vi "Datacluster manually remove bad data pts.vi"(10 "Datasets to be processed":T2(array[cluster]), 11 "data cluster":cluster{"all rows":dbl[][]}[](array[cluster])) -> (3 "data cluster out":cluster{"all rows":dbl[][]}[](array[cluster]))   [LabVIEW 2021]
panel:
  in  "selected XY data":dbl[][](array[numeric])
  in  "operation":enum16{"keep pts", "delete pts", "move pts"}(ring)=enum."delete pts"
  in  "start over":bool
  in  "auto scale once":bool
  in  "Do not Save and Proceed":bool
  in  "reset cursors":bool
  out "String":string="KR6_Rh3In3Ge4"
  in  "Undo":bool
  in  "Save and Proceed":bool
  in  "data selection mode":T1(ring)
  in  "Update":bool
  out "XY Graph":cluster{"x-array":dbl[], "y-array":dbl[]}(graph)
  # "Caution: All rows will be affected."
  # "Operation\ndelete/keep data pts: selected data pts will be removed or kept.\nmove data pts: (1) use zoom/drag selection mode (2) type in data"
  # "Remove pts"
  # "(4) Start processing"
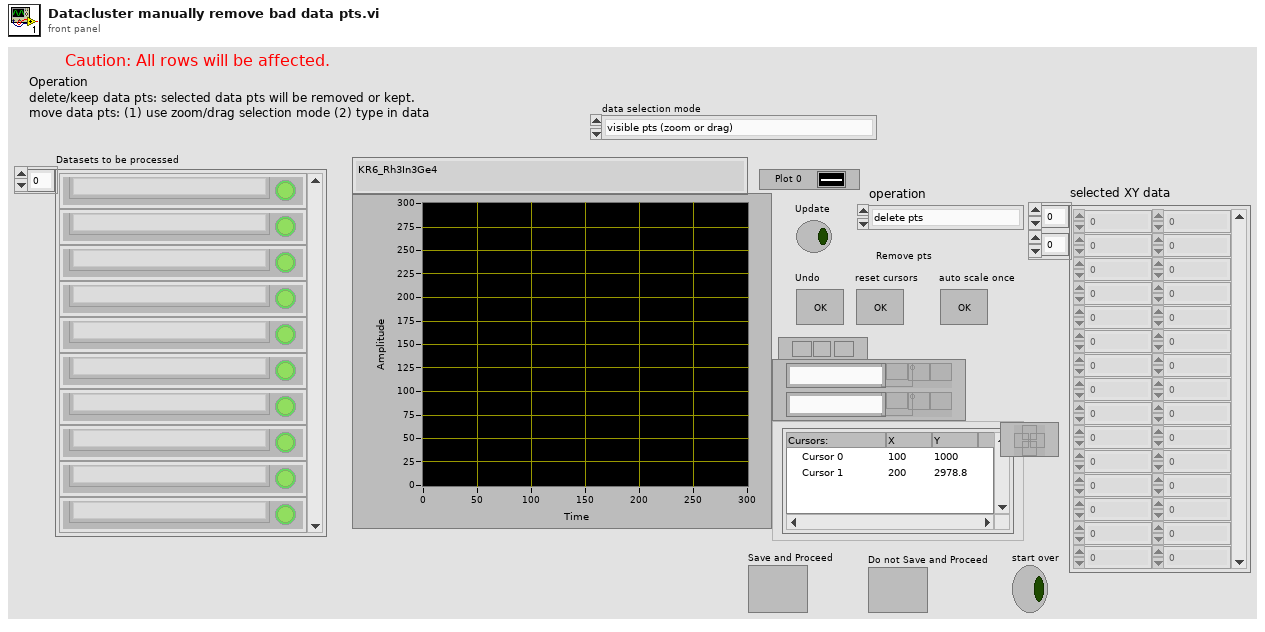
[diagram p1: front panel]
types:
  T1 = enum16{"visible pts (zoom or drag)", "pts inside the rectangle defined by the cursors", "pts between two horizontal cursors", "pts between two vertical cursor lines"}
  T2 = cluster{"String":string, "Boolean":bool, "begin":u32, "length":u32, "y weight":dbl}[]
  T3 = enum16{"no change", "show whole data", "show whole panel"}
  T4 = enum16{"no change", "no auto", "auto once", "auto"}
  T5 = enum16{"no change", "move to data center", "move to data corner", "move to panel center", "move to panel corner"}
  T6 = enum16{"no change", "hide cursor", "cross", "horizontal", "vertical"}
  T7 = enum16{"visible pts (use zoom or drag)", "pts inside rectangle defined the cursor lines", "pts between two horizontal cursors", "pts between two vertical cursor lines"}
  T8 = typedef "LVCursorListTypeDef.ctl" = cluster{"Name":string, "Color":u32, "Style":u8, "Point Style":u8, "Name Visible":bool, "Allow Drag":bool, "Cursor Mode":u32, "Plot":i32, "Index":i32, "Position":cluster{"X":dbl, "Y":dbl}, "X Scale":u32, "Y Scale":u32, "Watch Plots":i32[], "Watch All Plots":bool, "Plot Area":i32, "Label Offset":cluster{"X":dbl, "Y":dbl}}[]
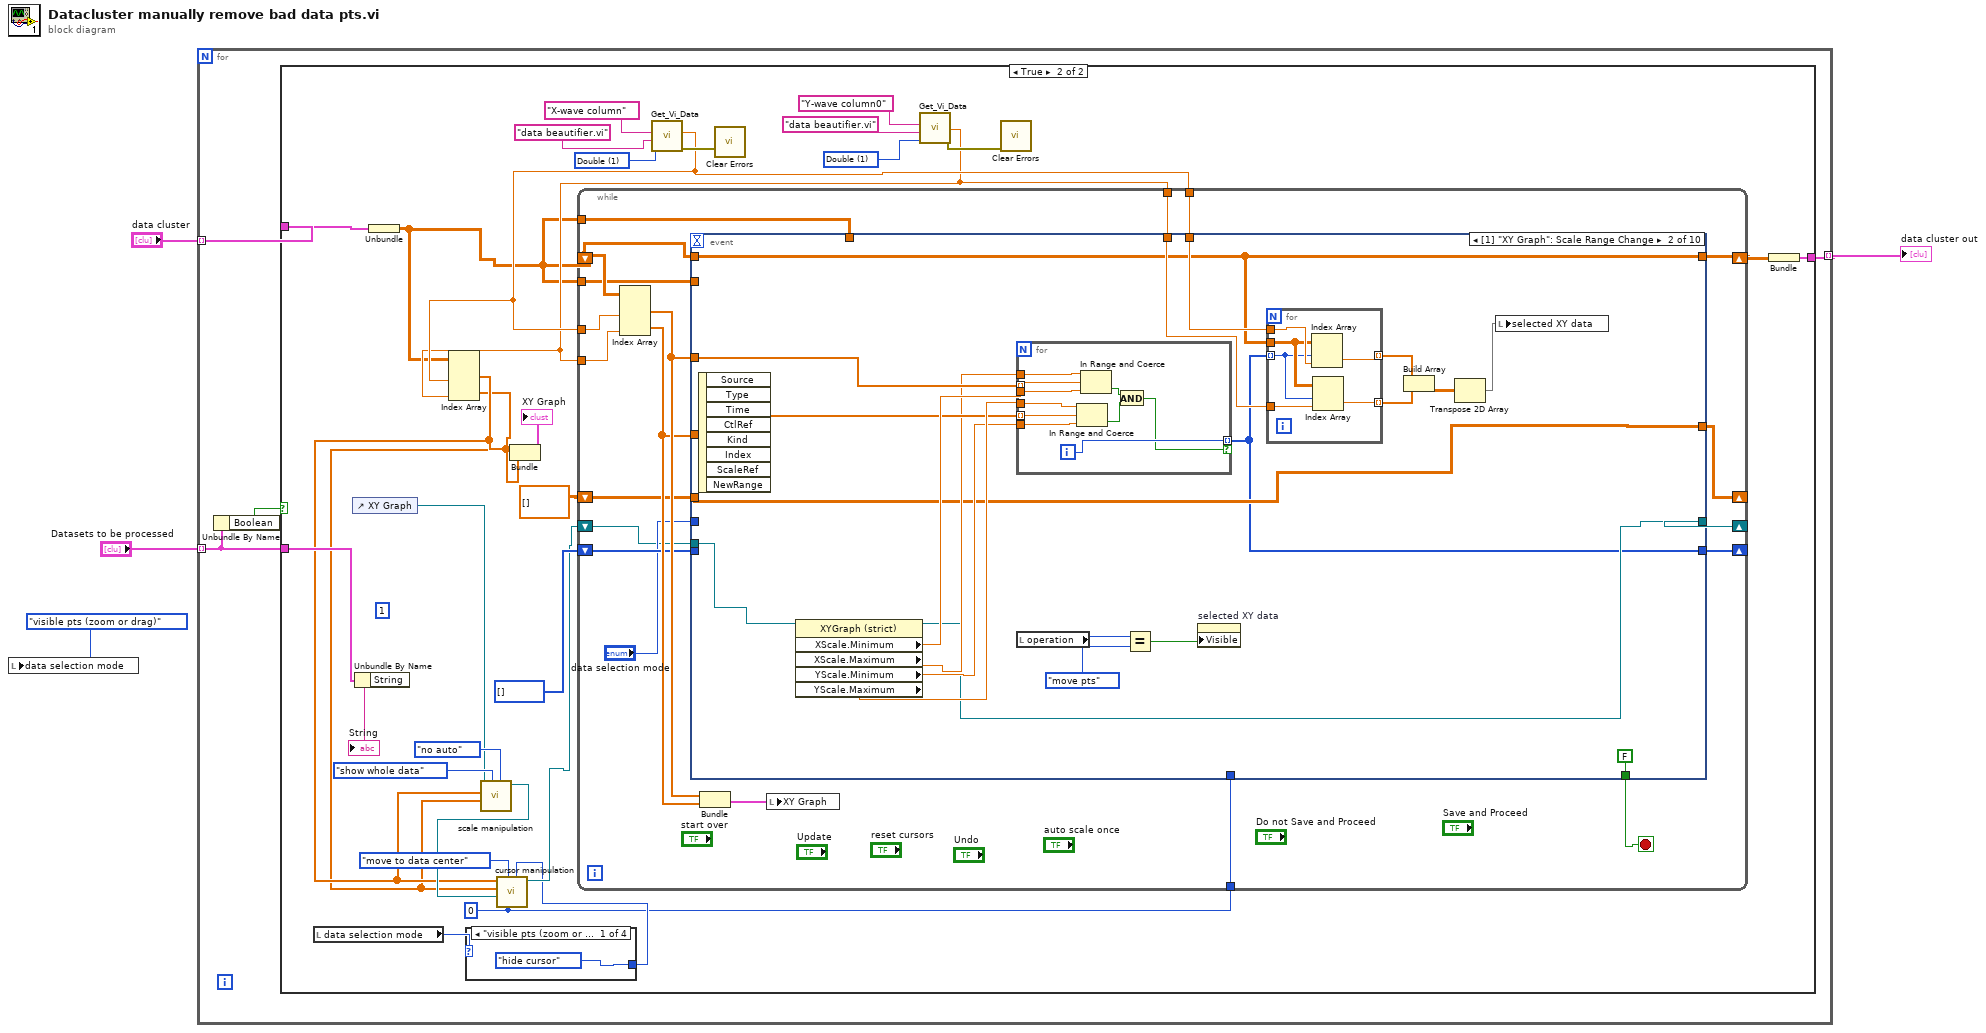
[diagram p0: block diagram]
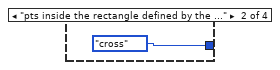
[diagram p3: hidden frame]
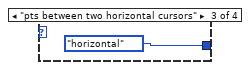
[diagram p4: hidden frame]
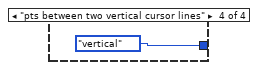
[diagram p5: hidden frame]
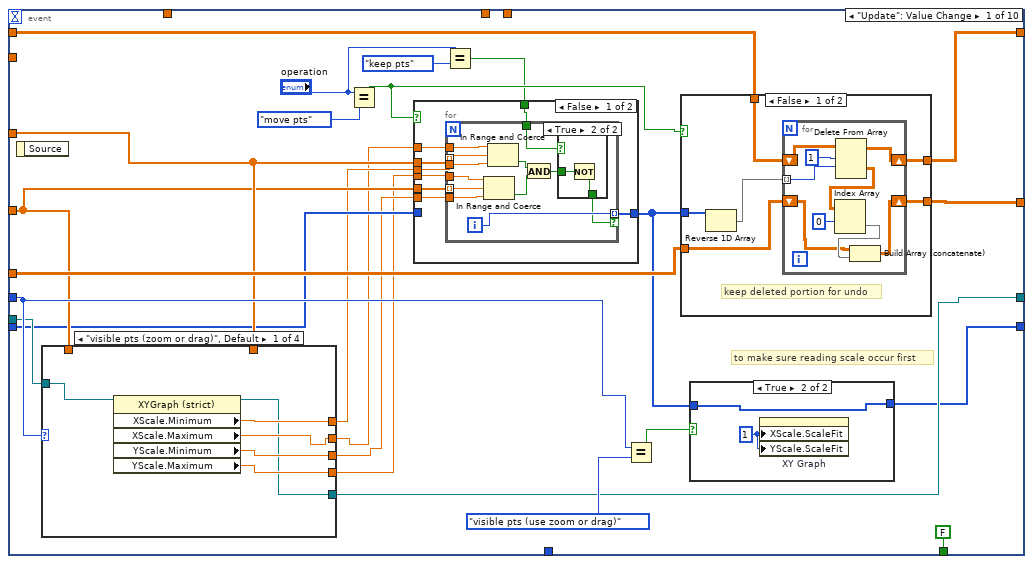
[diagram p6: hidden frame]
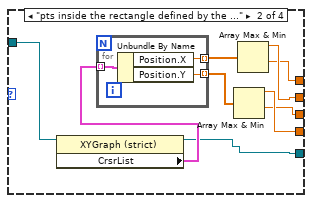
[diagram p11: hidden frame]
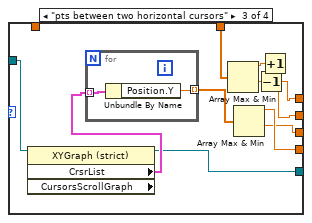
[diagram p12: hidden frame]
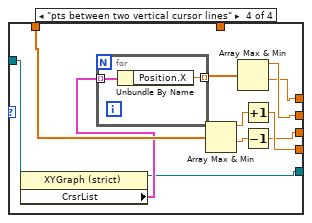
[diagram p13: hidden frame]
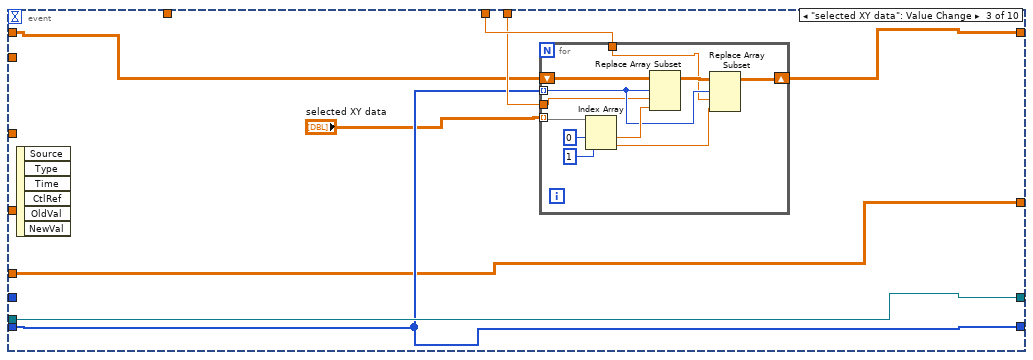
[diagram p14: hidden frame]
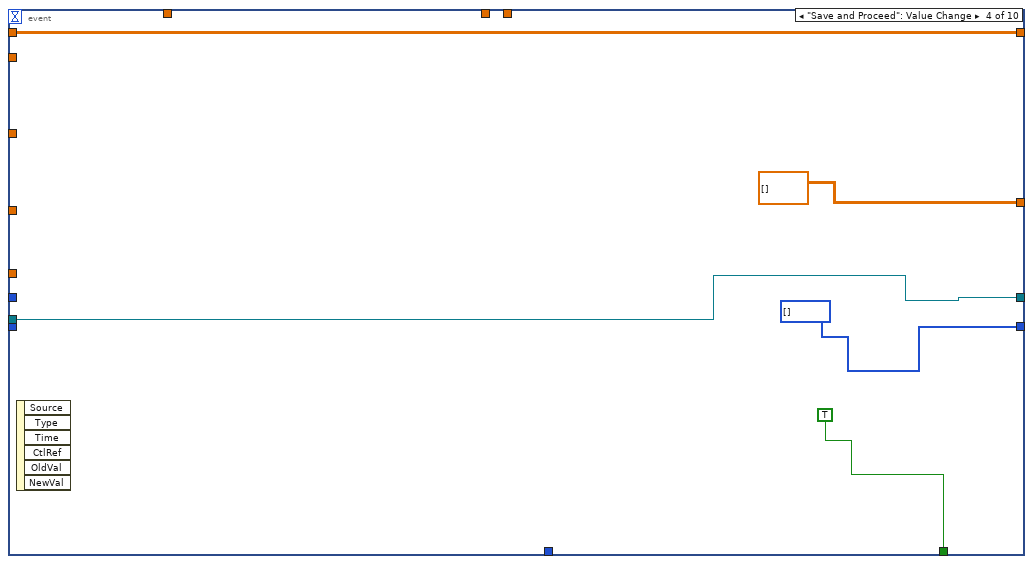
[diagram p15: hidden frame]
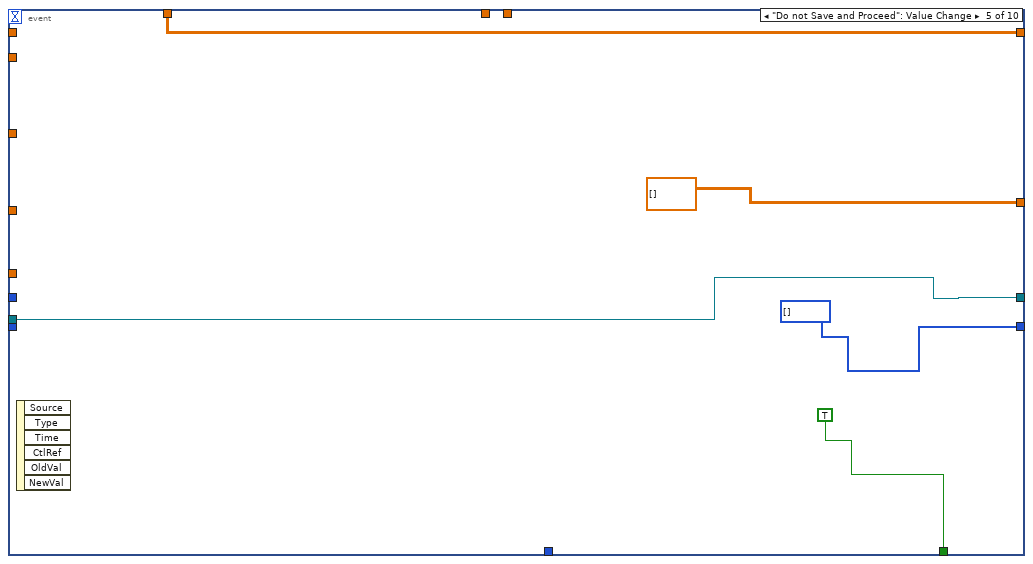
[diagram p16: hidden frame]
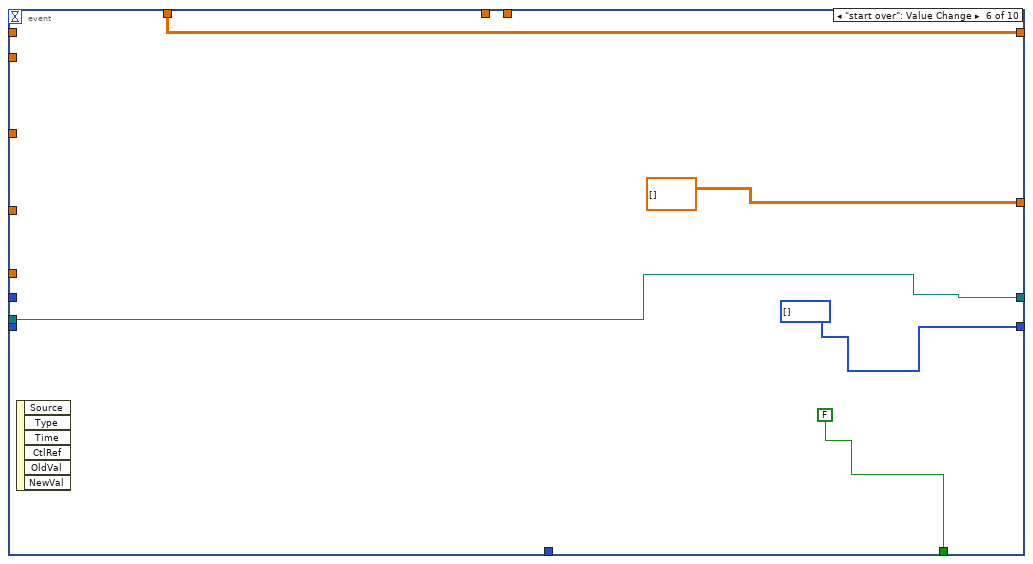
[diagram p17: hidden frame]
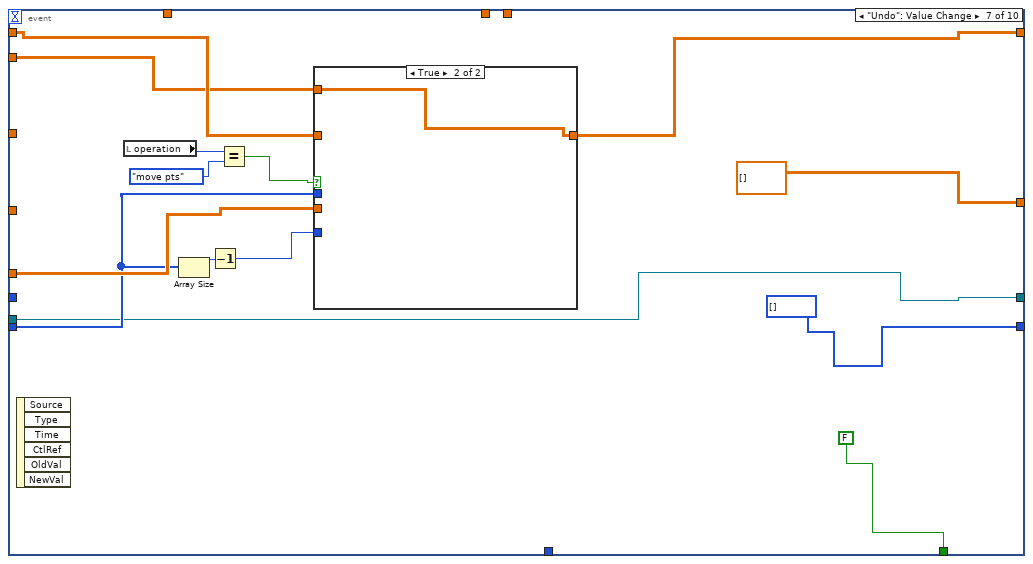
[diagram p18: hidden frame]
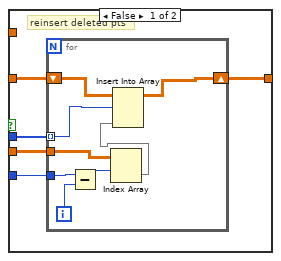
[diagram p19: hidden frame]
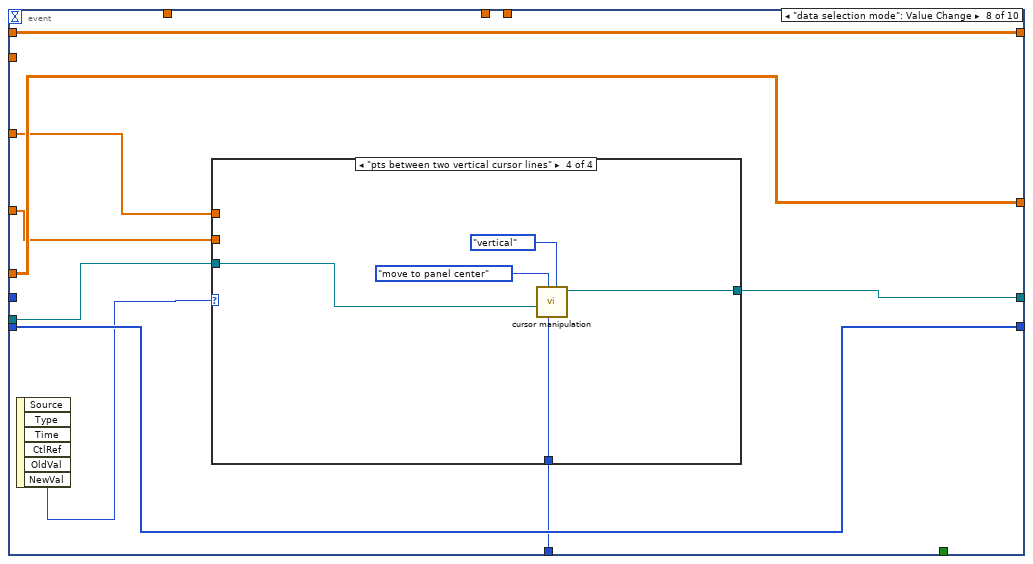
[diagram p20: hidden frame]
diagram:
  n1 = local write "data selection mode"(T1."visible pts (zoom or drag)" ("data selection mode")) -> ()
  n2 = for {
    tunnel: "Datasets to be processed" -> [w6] mode=indexing
    tunnel: "data cluster" -> [w8] mode=indexing
    tunnel: [w7] -> w2 mode=indexing
    n3 = Unbundle By Name(w6) -> ("Boolean"=w5:bool)
    n4 = case shown="True" w5 {
      tunnel: w6 -> [_ w27]
      tunnel: w8 -> [w9 w26]
      tunnel: [w9 w25] -> w7
      frame False {
      }
      frame True {
        w14 = u32 0 ("Cursor.Cursor Mode")
        (unwired) u8 1 ("X Scale.Scale Fit")
        w33 = u16 1 items=["String", "Double", "Boolean", "Variant"] ("Data Type")
        w36 = u16 1 items=["String", "Double", "Boolean", "Variant"] ("Data Type")
        n5 = local read "data selection mode"() -> (w16:T1)
        n6 = control-ref of="XY Graph"() -> (w17:refnum<vi>)
        n7 = Unbundle By Name(w27) -> ("String"=→"String":string)
        n8 = Unbundle(w26) -> ("all rows"=w10:dbl[][])
        n9 = case shown="\"visible pts (zoom or drag)\", Default" w16 {
          tunnel: [T6."hide cursor" ("cursor type") T6."cross" ("cursor type") T6."horizontal" ("cursor type") T6."vertical" ("cursor type")] -> w15
          frame "visible pts (zoom or drag)", Default {
          }
          frame "pts inside the rectangle defined by the cursors" {
          }
          frame "pts between two horizontal cursors" {
          }
          frame "pts between two vertical cursor lines" {
          }
        }
        n10 = call "Get_Vi_Data.vi"("Data Type"=w36, "VI name"="data beautifier.vi", "Control Name"="X-wave column") -> ("error out"=w35:errorcluster, "Data (Double)"=w12:dbl)  [unwired: 4 in, 3 out]
        n11 = call <vilib>:"Clear Errors.vi"("error in (no error)"=w35) -> ()  [unwired: 5 in, 2 out]
        n12 = call "Get_Vi_Data.vi"("Data Type"=w33, "VI name"="data beautifier.vi", "Control Name"="Y-wave column0") -> ("error out"=w31:errorcluster, "Data (Double)"=w11:dbl)  [unwired: 4 in, 3 out]
        n13 = Index Array(array=w10, index (col) #1=w12, index (col) #2=w11) -> (element #1=w19:dbl[], element #2=w18:dbl[])  [unwired: 2 in]
        n14 = call "scale manipulation.vi"("scale fit"=T4."no auto", "rescale"=T3."show whole data", "y-array"=w18, "x-array"=w19, "graph reference in"=w17) -> ("reference out"=w22:refnum<vi>)  [unwired: 6 in]
        n15 = call "cursor manipulation.vi"("cursor type"=w15, "Cursor.Cursor Mode"=w14, "cursor position"=T5."move to data center" ("mode"), "graph reference in"=w22, "y-array"=w18, "x-array"=w19) -> ("reference out"=w21:refnum<vi>)  [unwired: 5 in]
        n16 = Bundle("all rows"=w19, "all rows"=w18) -> (→"XY Graph":cluster{"all rows":dbl[], "all rows":dbl[]})  [unwired: 1 in]
        n17 = while {
          tunnel: w12 -> [w47]
          tunnel: w11 -> [w54]
          shift-right: [w60] -> w39
          shift-left: w10 -> [w61]
          shift-right: [w57] -> _
          shift-left: dbl[][] [] -> [w58]
          shift-right: [w56] -> _
          shift-left: i32[] [] -> [w55]
          tunnel: w10 -> [w52]
          tunnel: w14 -> [w49]
          shift-right: [w48] -> _
          shift-left: w21 -> [w51]
          tunnel: w12 -> [w46]
          tunnel: w11 -> [w45]
          tunnel: w10 -> [w44]
          stop <- w59 stop-if-true
          n18 = Index Array(array=w61, index (col) #1=w47, index (col) #2=w54) -> (element #1=w63:dbl[], element #2=w62:dbl[])  [unwired: 2 in]
          n19 = event shown="[1] \"XY Graph\": Scale Range Change" {
            selector: _ -> [_ _ _ _ _ _ _ _ _ _]
            dyn-events: _ -> [_ _ _ _ _ _ _ _ _ _]
            timeout: _ -> [_ _ _ _ _ _ _ _ _ _]
            tunnel: w63 -> [w79 w192 _ _ _ _ _ w279 _ w314]
            tunnel: w62 -> [w78 w191 _ _ _ _ _ w278 _ w313]
            tunnel: w61 -> [w87 w183 w215 w236 _ _ w260 w280 w309 w318]
            tunnel: [w86 w183 w218 w236 w239 w244 w254 w280 w309 w318] -> w60
            tunnel: [FALSE FALSE _ TRUE TRUE FALSE FALSE _ _ _] -> w59
            tunnel: [w84 w182 w214 dbl[][] [] dbl[][] [] dbl[][] [] dbl[][] [] w283 w311 w320] -> w57
            tunnel: w58 -> [w83 w182 w214 _ _ _ w259 w283 w311 w320]
            tunnel: [w65 w180 w216 i32[] [] i32[] [] i32[] [] i32[] [] w282 w310 w319] -> w56
            tunnel: w55 -> [w70 _ w216 _ _ _ w257 w282 w310 w319]
            tunnel: "data selection mode" -> [w82 _ _ _ _ _ _ _ _ _]
            tunnel: w52 -> [_ _ _ _ w239 w244 _ _ _ _]
            tunnel: w51 -> [w72 w189 w217 w232 w237 w242 w251 w277 w308 w317]
            tunnel: w49 -> [_ _ _ _ _ _ _ w276 w305 _]
            tunnel: [w71 w188 w217 w232 w237 w242 w251 w275 w304 w312] -> w48
            tunnel: w46 -> [_ w187 w219 _ _ _ _ _ _ _]
            tunnel: w45 -> [_ w186 w220 _ _ _ _ _ _ _]
            tunnel: w44 -> [_ _ _ _ _ _ w247 _ _ _]
            event "Update": Value Change {
              # "to make sure reading scale occur first"
              n20 = event-data() -> ()  [unwired: 1 in, 1 out]
              n21 = case shown="\"visible pts (zoom or drag)\", Default" w82 {
                tunnel: [w133 w142 w157 w167] -> w66
                tunnel: [w134 w141 w156 w166] -> w67
                tunnel: [w136 w143 w153 w171] -> w69
                tunnel: [w135 w144 w154 w172] -> w68
                tunnel: w79 -> [_ _ w155 _]
                tunnel: w78 -> [_ _ _ w168]
                tunnel: w72 -> [w137 w140 w152 w165]
                tunnel: [w132 w138 w150 w163] -> w71
                frame "visible pts (zoom or drag)", Default {
                  n22 = property class="XYGraph (strict)"(reference=w137) -> (reference out=w132:refnum<vi>, "XScale.Minimum"=w136:dbl, "XScale.Maximum"=w135:dbl, "YScale.Minimum"=w134:dbl, "YScale.Maximum"=w133:dbl)  [unwired: 1 in, 1 out]
                }
                frame "pts inside the rectangle defined by the cursors" {
                  n23 = property class="XYGraph (strict)"(reference=w140) -> (reference out=w138:refnum<vi>, "CrsrList"=w139:T8)  [unwired: 1 in, 1 out]
                  n24 = for {
                    tunnel: w139 -> [w149] mode=indexing
                    tunnel: [w148] -> w146 mode=indexing
                    tunnel: [w147] -> w145 mode=indexing
                    n25 = Unbundle By Name(w149) -> ("Position.X"=w148:dbl, "Position.Y"=w147:dbl)
                  }
                  n26 = Array Max & Min(array=w145) -> (max value=w142:dbl, min value=w141:dbl)  [unwired: 2 out]
                  n27 = Array Max & Min(array=w146) -> (max value=w144:dbl, min value=w143:dbl)  [unwired: 2 out]
                }
                frame "pts between two horizontal cursors" {
                  n28 = property class="XYGraph (strict)" props=["CrsrList", "CursorsScrollGraph"](reference=w152) -> (reference out=w150:refnum<vi>, "CrsrList"=w151:T8)  [unwired: 1 in, 2 out]
                  n29 = for {
                    tunnel: [w162] -> w160 mode=indexing
                    tunnel: w151 -> [w161] mode=indexing
                    n30 = Unbundle By Name(w161) -> ("Position.Y"=w162:dbl)
                  }
                  n31 = Array Max & Min(array=w155) -> (max value=w159:dbl, min value=w158:dbl)  [unwired: 2 out]
                  n32 = Array Max & Min(array=w160) -> (max value=w157:dbl, min value=w156:dbl)  [unwired: 2 out]
                  n33 = Decrement(x=w158) -> (x-1=w153:dbl)
                  n34 = Increment(x=w159) -> (x+1=w154:dbl)
                }
                frame "pts between two vertical cursor lines" {
                  n35 = property class="XYGraph (strict)"(reference=w165) -> (reference out=w163:refnum<vi>, "CrsrList"=w164:T8)  [unwired: 1 in, 1 out]
                  n36 = for {
                    tunnel: w164 -> [w175] mode=indexing
                    tunnel: [w174] -> w173 mode=indexing
                    n37 = Unbundle By Name(w175) -> ("Position.X"=w174:dbl)
                  }
                  n38 = Array Max & Min(array=w168) -> (max value=w170:dbl, min value=w169:dbl)  [unwired: 2 out]
                  n39 = Array Max & Min(array=w173) -> (max value=w172:dbl, min value=w171:dbl)  [unwired: 2 out]
                  n40 = Increment(x=w170) -> (x+1=w167:dbl)
                  n41 = Decrement(x=w169) -> (x-1=w166:dbl)
                }
              }
              n42 = Equal?(x="operation", y=enum16{"keep pts", "delete pts", "move pts"}."move pts") -> (x = y?=w76:bool)
              n43 = Equal?(x="operation", y=enum16{"keep pts", "delete pts", "move pts"}."keep pts") -> (x = y?=w73:bool)
              n44 = case shown="False" w76 {
                tunnel: w66 -> [w95 _]
                tunnel: w67 -> [w94 _]
                tunnel: w69 -> [w93 _]
                tunnel: [w92 w111] -> w64
                tunnel: w79 -> [w91 _]
                tunnel: w78 -> [w90 _]
                tunnel: w73 -> [w89 _]
                tunnel: w68 -> [w88 _]
                tunnel: w70 -> [_ w111]
                frame False {
                  n45 = for {
                    tunnel: w91 -> [w107] mode=indexing
                    tunnel: w90 -> [w103] mode=indexing
                    tunnel: w95 -> [w102]
                    tunnel: [w104] -> w92 mode=indexing if=w96
                    tunnel: w94 -> [w101]
                    tunnel: w88 -> [w100]
                    tunnel: w93 -> [w99]
                    tunnel: w89 -> [w98]
                    i -> [w104]
                    n46 = In Range and Coerce(upper limit=w102, x=w103, lower limit=w101) -> (In Range?=w106:bool)  [unwired: 1 out]
                    n47 = In Range and Coerce(upper limit=w100, x=w107, lower limit=w99) -> (In Range?=w105:bool)  [unwired: 1 out]
                    n48 = And(x=w105, y=w106) -> (x .and. y?=w97:bool)
                    n49 = case shown="True" w98 {
                      tunnel: w97 -> [w108 w110]
                      tunnel: [w108 w109] -> w96
                      frame False {
                      }
                      frame True {
                        n50 = Not(x=w110) -> (.not. x?=w109:bool)
                      }
                    }
                  }
                }
                frame True {
                }
              }
              n51 = Equal?(x=w82, y=T7."visible pts (use zoom or drag)") -> (x = y?=w80:bool)
              n52 = case shown="False" w76 {
                tunnel: w87 -> [w117 w128]
                tunnel: [w116 w128] -> w86
                tunnel: [w115 w127] -> w84
                tunnel: w83 -> [w113 w127]
                tunnel: w64 -> [w112 _]
                frame False {
                  # "keep deleted portion for undo"
                  n53 = Reverse 1D Array(array=w112) -> (reversed array=w114:i32[])
                  n54 = for {
                    tunnel: w114 -> [w125] mode=indexing
                    shift-right: [w126] -> w116
                    shift-left: w117 -> [w123]
                    shift-right: [w119] -> w115
                    shift-left: w113 -> [w118]
                    n55 = Delete From Array(array=w123, length=1, index (row)=w125) -> (deleted portion=w122:dbl[][], array with subset deleted=w126:dbl[][])  [unwired: 1 in]
                    n56 = Index Array(array=w122, index (row)=0) -> (element=w120:dbl[])  [unwired: 1 in]
                    n57 = Build Array (concatenate)(w118, w120) -> (w119:dbl[][])
                  }
                }
                frame True {
                }
              }
              n58 = case shown="True" w80 {
                tunnel: [w129 w130] -> w65
                tunnel: w64 -> [w129 w130]
                frame False {
                }
                frame True {
                  w131 = u8 1 ("X Scale.Scale Fit")
                  n59 = property on="XY Graph" class="XYGraph (strict)"("XScale.ScaleFit"=w131, "YScale.ScaleFit"=w131) -> ()  [unwired: 2 in, 2 out]
                }
              }
            }
            event "XY Graph": Scale Range Change {
              n60 = event-data() -> ()  [unwired: 1 in, 8 out]
              n61 = property class="XYGraph (strict)"(reference=w189) -> (reference out=w188:refnum<vi>, "XScale.Minimum"=w194:dbl, "XScale.Maximum"=w190:dbl, "YScale.Minimum"=w195:dbl, "YScale.Maximum"=w196:dbl)  [unwired: 1 in, 1 out]
              n62 = for {
                tunnel: w192 -> [w212] mode=indexing
                tunnel: w191 -> [w208] mode=indexing
                tunnel: w196 -> [w207]
                tunnel: [w209] -> w180 mode=indexing if=w203
                tunnel: w195 -> [w206]
                tunnel: w190 -> [w205]
                tunnel: w194 -> [w204]
                i -> [w209]
                n63 = In Range and Coerce(upper limit=w207, x=w208, lower limit=w206) -> (In Range?=w211:bool)  [unwired: 1 out]
                n64 = In Range and Coerce(upper limit=w205, x=w212, lower limit=w204) -> (In Range?=w210:bool)  [unwired: 1 out]
                n65 = And(x=w210, y=w211) -> (x .and. y?=w203:bool)
              }
              n66 = local read "operation"() -> (w179:enum16{"keep pts", "delete pts", "move pts"})
              n67 = Equal?(x=w179, y=enum16{"keep pts", "delete pts", "move pts"}."move pts" ("operation")) -> (x = y?=w176:bool)
              n68 = property on="selected XY data" class="Arr (strict)"("Visible"=w176) -> ()  [unwired: 2 in, 2 out]
              n69 = for {
                tunnel: w180 -> [w200] mode=indexing
                tunnel: w183 -> [w201]
                tunnel: w187 -> [w202]
                tunnel: w186 -> [w199]
                tunnel: [w198] -> w185 mode=indexing
                tunnel: [w197] -> w184 mode=indexing
                n70 = Index Array(array=w201, index (row)=w200, index (col)=w202) -> (element=w198:dbl)
                n71 = Index Array(array=w201, index (row)=w200, index (col)=w199) -> (element=w197:dbl)
              }
              n72 = Build Array(w185, w184) -> (w181:dbl[][])
              n73 = Transpose 2D Array(2D array=w181) -> (transposed array=w177:dbl[][])
              n74 = local write "selected XY data"(w177) -> ()
            }
            event "selected XY data": Value Change {
              n75 = event-data() -> ()  [unwired: 1 in, 6 out]
              n76 = for {
                tunnel: w216 -> [w225] mode=indexing
                tunnel: w220 -> [w221]
                tunnel: "selected XY data" -> [w230] mode=indexing
                shift-right: [w223] -> w218
                shift-left: w215 -> [w231]
                tunnel: w219 -> [w222]
                n77 = Index Array(array=w230, index #1=0 ("index"), index #2=1 ("index")) -> (element #1=w227:dbl, element #2=w224:dbl)
                n78 = Replace Array Subset(array=w231, new element=w227, index (row)=w225, index (col)=w222) -> (w226:dbl[][])
                n79 = Replace Array Subset(array=w226, new element=w224, index (row)=w225, index (col)=w221) -> (w223:dbl[][])
              }
            }
            event "Save and Proceed": Value Change {
              n80 = event-data() -> ()  [unwired: 1 in, 6 out]
            }
            event "Do not Save and Proceed": Value Change {
              n81 = event-data() -> ()  [unwired: 1 in, 6 out]
            }
            event "start over": Value Change {
              n82 = event-data() -> ()  [unwired: 1 in, 6 out]
            }
            event "Undo": Value Change {
              n83 = event-data() -> ()  [unwired: 1 in, 6 out]
              n84 = local read "operation"() -> (w250:enum16{"keep pts", "delete pts", "move pts"})
              n85 = Array Size(array=w257) -> (size(s)=w258:i32)
              n86 = Decrement(x=w258) -> (x-1=w256:i32)
              n87 = Equal?(x=w250, y=enum16{"keep pts", "delete pts", "move pts"}."move pts" ("operation")) -> (x = y?=w248:bool)
              n88 = case shown="True" w248 {
                tunnel: w260 -> [w265 _]
                tunnel: w259 -> [w264 _]
                tunnel: w257 -> [w263 _]
                tunnel: w256 -> [w262 _]
                tunnel: [w261 w274] -> w254
                tunnel: w247 -> [_ w274]
                frame False {
                  # "reinsert deleted pts"
                  n89 = for {
                    tunnel: w263 -> [w272] mode=indexing
                    shift-right: [w271] -> w261
                    shift-left: w265 -> [w273]
                    tunnel: w264 -> [w270]
                    tunnel: w262 -> [w269]
                    i -> [w267]
                    n90 = Subtract(x=w269, y=w267) -> (x-y=w268:i32)
                    n91 = Index Array(array=w270, index (row)=w268) -> (element=w266:dbl[])  [unwired: 1 in]
                    n92 = Insert Into Array(array=w273, index (row)=w272, new element=w266) -> (w271:dbl[][])  [unwired: 1 in]
                  }
                }
                frame True {
                }
              }
            }
            event "data selection mode": Value Change {
              n93 = event-data() -> ("NewVal"=w281:T1)  [unwired: 1 in, 5 out]
              n94 = case shown="\"pts between two vertical cursor lines\"" w281 {
                tunnel: w279 -> [_ _ _ _]
                tunnel: w278 -> [_ _ _ _]
                tunnel: w277 -> [w288 w291 w296 w301]
                tunnel: w276 -> [w285 w290 w295 w300]
                tunnel: [w284 w289 w294 w299] -> w275
                frame "visible pts (zoom or drag)", Default {
                  n95 = call "cursor manipulation.vi"("cursor type"=T6."hide cursor", "Cursor.Cursor Mode"=w285, "cursor position"=T5."no change" ("mode"), "graph reference in"=w288) -> ("reference out"=w284:refnum<vi>)  [unwired: 7 in]
                }
                frame "pts between two horizontal cursors" {
                  n96 = call "cursor manipulation.vi"("cursor type"=T6."horizontal", "Cursor.Cursor Mode"=w290, "cursor position"=T5."move to panel center" ("mode"), "graph reference in"=w291) -> ("reference out"=w289:refnum<vi>)  [unwired: 7 in]
                }
                frame "pts inside the rectangle defined by the cursors" {
                  n97 = call "cursor manipulation.vi"("cursor type"=T6."cross", "Cursor.Cursor Mode"=w295, "cursor position"=T5."move to panel center" ("mode"), "graph reference in"=w296) -> ("reference out"=w294:refnum<vi>)  [unwired: 7 in]
                }
                frame "pts between two vertical cursor lines" {
                  n98 = call "cursor manipulation.vi"("cursor type"=T6."vertical", "Cursor.Cursor Mode"=w300, "cursor position"=T5."move to panel center" ("mode"), "graph reference in"=w301) -> ("reference out"=w299:refnum<vi>)  [unwired: 7 in]
                }
              }
            }
            event "reset cursors": Value Change {
              n99 = event-data() -> ()  [unwired: 1 in, 6 out]
              n100 = call "cursor manipulation.vi"("cursor type"=T6."no change", "Cursor.Cursor Mode"=w305, "cursor position"=T5."move to panel center", "graph reference in"=w308) -> ("reference out"=w304:refnum<vi>)  [unwired: 7 in]
            }
            event "auto scale once": Value Change {
              n101 = event-data() -> ()  [unwired: 1 in, 6 out]
              n102 = call "scale manipulation.vi"("scale fit"=T4."no auto", "rescale"=T3."show whole data", "y-array"=w313, "x-array"=w314, "graph reference in"=w317) -> ("reference out"=w312:refnum<vi>)  [unwired: 6 in]
            }
          }
          n103 = Bundle("all rows"=w63, "all rows"=w62) -> (w50:cluster{"all rows":dbl[], "all rows":dbl[]})  [unwired: 1 in]
          n104 = local write "XY Graph"(w50) -> ()
        }
        n105 = call <vilib>:"Clear Errors.vi"("error in (no error)"=w31) -> ()  [unwired: 5 in, 2 out]
        n106 = Bundle("all rows"=w39) -> (w25:cluster{"all rows":dbl[][]})  [unwired: 1 in]
      }
    }
  }
  "data cluster out" <- w2
